vi "get_accuracy.vi"(1 "predict":dbl[][](array[numeric]), 2 "Y":dbl[](array[numeric])) -> (0 "accuracy":dbl)   [LabVIEW 2023]
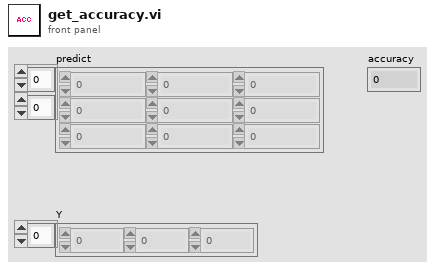
[diagram p1: front panel]
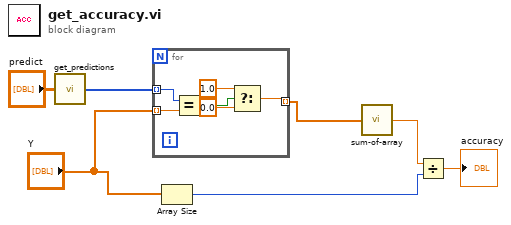
[diagram p0: block diagram]
diagram:
  n1 = call "get_predictions.vi"("2D array"="predict") -> ("Array"=w2:i32[])
  n2 = for {
    tunnel: w2 -> [w13] mode=indexing
    tunnel: "Y" -> [w12] mode=indexing
    tunnel: [w8] -> w4 mode=indexing
    n3 = Equal?(x=w13, y=w12) -> (x = y?=w11:bool)
    n4 = Select(t=1.0, s=w11, f=0.0) -> (s? t:f=w8:dbl)
  }
  n5 = Array Size(array="Y") -> (size(s)=w6:i32)
  n6 = call "sum-of-array.vi"("Array"=w4) -> ("sum of array"=w5:dbl)
  n7 = Divide(x=w5, y=w6) -> (x/y=→"accuracy":dbl)
